vi "Get Array Values (Boolean[]).vi"(8 "error in (no error)":errorcluster, 11 "JSON Value in":refnum<class "JSON Value.lvclass">) -> (0 "error out":errorcluster, 3 "values":bool[](array[boolean]))   [LabVIEW 2016, in "JSON Value.lvclass"]
doc: "Returns the element type of each element in a JSON Array. If all elements are of the same type, single type is true."
uses:
  JSON Value.lvclass
  JSON Types.ctl
  subVIs/Errors.ctl
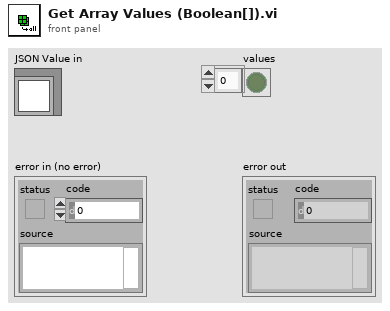
[diagram p1: front panel]
types:
  T1 = typedef "JSON Value.lvclass/JSON Types.ctl" = enum8{"String", "Numeric", "Boolean", "NULL", "Object", "Array"}
  T2 = typedef "JSON Value.lvclass/Errors.ctl" = enum8{"No key", "Key path type", "Array OOB", "Type Mismatch", "Invalid Token"}
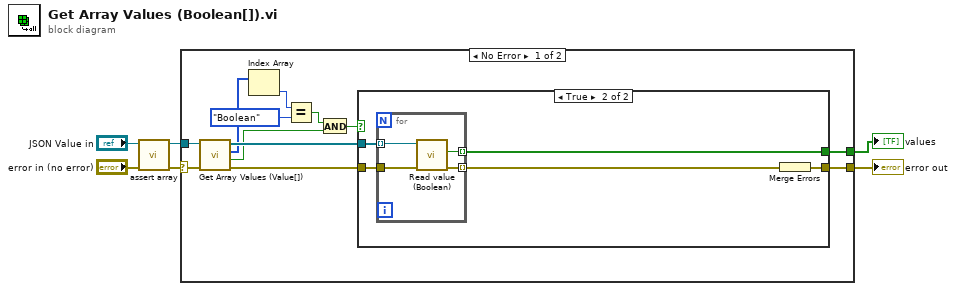
[diagram p0: block diagram]
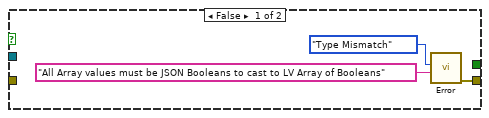
[diagram p2: hidden frame]
diagram:
  n1 = call "assert array.vi"("error in (no error)"="error in (no error)", "JSON Value in"="JSON Value in") -> ("error out"=w3:errorcluster, "JSON Value out"=w1:refnum<class "JSON Value.lvclass">)  [unwired: 8 in]
  n2 = case shown="No Error" w3 {
    selector: w3 -> [w17 w31]
    tunnel: w1 -> [w18 _]
    tunnel: [w15 w31] -> w5
    tunnel: [w8 _] -> w4
    frame No Error {
      n3 = call "Get Array Values (Value[]).vi"("error in (no error)"=w17, "JSON Value in"=w18) -> ("error out"=w7:errorcluster, "single type?"=w10:bool, "types"=w14:T1[], "values"=w16:refnum<class "JSON Value.lvclass">[])  [unwired: 6 in]
      n4 = Index Array(array=w14) -> (element=w13:T1)  [unwired: 1 in]
      n5 = Equal?(x=w13, y=JSON_Types."Boolean") -> (x = y?=w11:bool)
      n6 = And(x=w11, y=w10) -> (x .and. y?=w9:bool)
      n7 = case shown="True" w9 {
        tunnel: w16 -> [_ w26]
        tunnel: [w19 w22] -> w15
        tunnel: [_ w25] -> w8
        tunnel: w7 -> [_ w23]
        frame False {
          n8 = call "Error.vi"("Data"="All Array values must be JSON Booleans to cast to LV Array of Booleans", "Error"=Errors."Type Mismatch") -> ("error out"=w19:errorcluster)  [unwired: 8 in]
        }
        frame True {
          n9 = for {
            tunnel: w26 -> [w27] mode=indexing
            tunnel: [w30] -> w25 mode=indexing
            tunnel: [w29] -> w24 mode=indexing
            tunnel: w23 -> [w28]
            n10 = call "Read value (Boolean).vi"("error in (no error)"=w28, "JSON Boolean in"=w27) -> ("error out"=w29:errorcluster, "value"=w30:bool)  [unwired: 7 in, 1 out]
          }
          n11 = Merge Errors(w24) -> (w22:errorcluster)
        }
      }
    }
    frame Error {
    }
  }
  "error out" <- w5
  "values" <- w4
